vi "Settings UI.vi"(10 "Alias":string, 11 "Init Settings In":T1={"Step Values"=[], "Only Execute When Test Running"=TRUE, "Reset Sequence When Test Starts"=TRUE, "Current Sequence ID"=0, "Total Iterations"=0, "Current Step Start Timestamp"=0.0, "Number of Sequence Steps"=0, "Num of Analog Channels"=0, "Num of Digital Channels"=0, "Delay Before Starting Sequence"=0.0, "Show UI"=FALSE, "Time Remaining"=0.0, "Test Running"=FALSE, "Pause Timestamp"=0.0, "Default Analog Values"=[], "Default Digital Values"=[]}) -> (2 "Applied Settings":T1={"Step Values"=[], "Only Execute When Test Running"=TRUE, "Reset Sequence When Test Starts"=TRUE, "Current Sequence ID"=0, "Total Iterations"=0, "Current Step Start Timestamp"=0.0, "Number of Sequence Steps"=0, "Num of Analog Channels"=0, "Num of Digital Channels"=0, "Delay Before Starting Sequence"=0.0, "Show UI"=FALSE, "Time Remaining"=0.0, "Test Running"=FALSE, "Pause Timestamp"=0.0, "Default Analog Values"=[], "Default Digital Values"=[]}, 3 "Show UI":bool)   [LabVIEW 2020, in "Sequencer with Output Values.lvlib" / "Sequencer with Output Values.lvclass"]
uses:
  Sequencer with Output Values.lvclass
  Params.ctl
  Step Settings.ctl
  Tree Manager/Tree Manager Mode.ctl
  Tree Manager/Control Refs.ctl
  Global Strings.vi
panel:
  in  "Tab Control":enum32{"Numeric", "String", "Bool", "Enum"}(tab)
  in  "Numeric":dbl min=1.0 max=100.0 step=1.0
  in  "String":string
  in  "Boolean":u16(ring) items=["False", "True"]
  in  "Ring":u16(ring) items=["Wait for end of step", "Repeat channel values"]
  in  "Plot Visible Array":cluster{"Boolean 2":bool}[](array[cluster]) caption="Show"
  in  "Applied Settings Control":T1={"Step Values"=[], "Only Execute When Test Running"=TRUE, "Reset Sequence When Test Starts"=TRUE, "Current Sequence ID"=0, "Total Iterations"=0, "Current Step Start Timestamp"=0.0, "Number of Sequence Steps"=0, "Num of Analog Channels"=0, "Num of Digital Channels"=0, "Delay Before Starting Sequence"=0.0, "Show UI"=FALSE, "Time Remaining"=0.0, "Test Running"=FALSE, "Pause Timestamp"=0.0, "Default Analog Values"=[], "Default Digital Values"=[]}
  out "Current Settings":T1={"Step Values"=[], "Only Execute When Test Running"=TRUE, "Reset Sequence When Test Starts"=TRUE, "Current Sequence ID"=0, "Total Iterations"=0, "Current Step Start Timestamp"=0.0, "Number of Sequence Steps"=0, "Num of Analog Channels"=0, "Num of Digital Channels"=0, "Delay Before Starting Sequence"=0.0, "Show UI"=FALSE, "Time Remaining"=0.0, "Test Running"=FALSE, "Pause Timestamp"=0.0, "Default Analog Values"=[], "Default Digital Values"=[]}
  in  "Close":bool
  in  "Apply":bool
  out "Channel Values Preview":waveform(dbl)[](graph)
  out "Setting Description":string
  in  "Settings Tree":string(tree) caption="Settings"
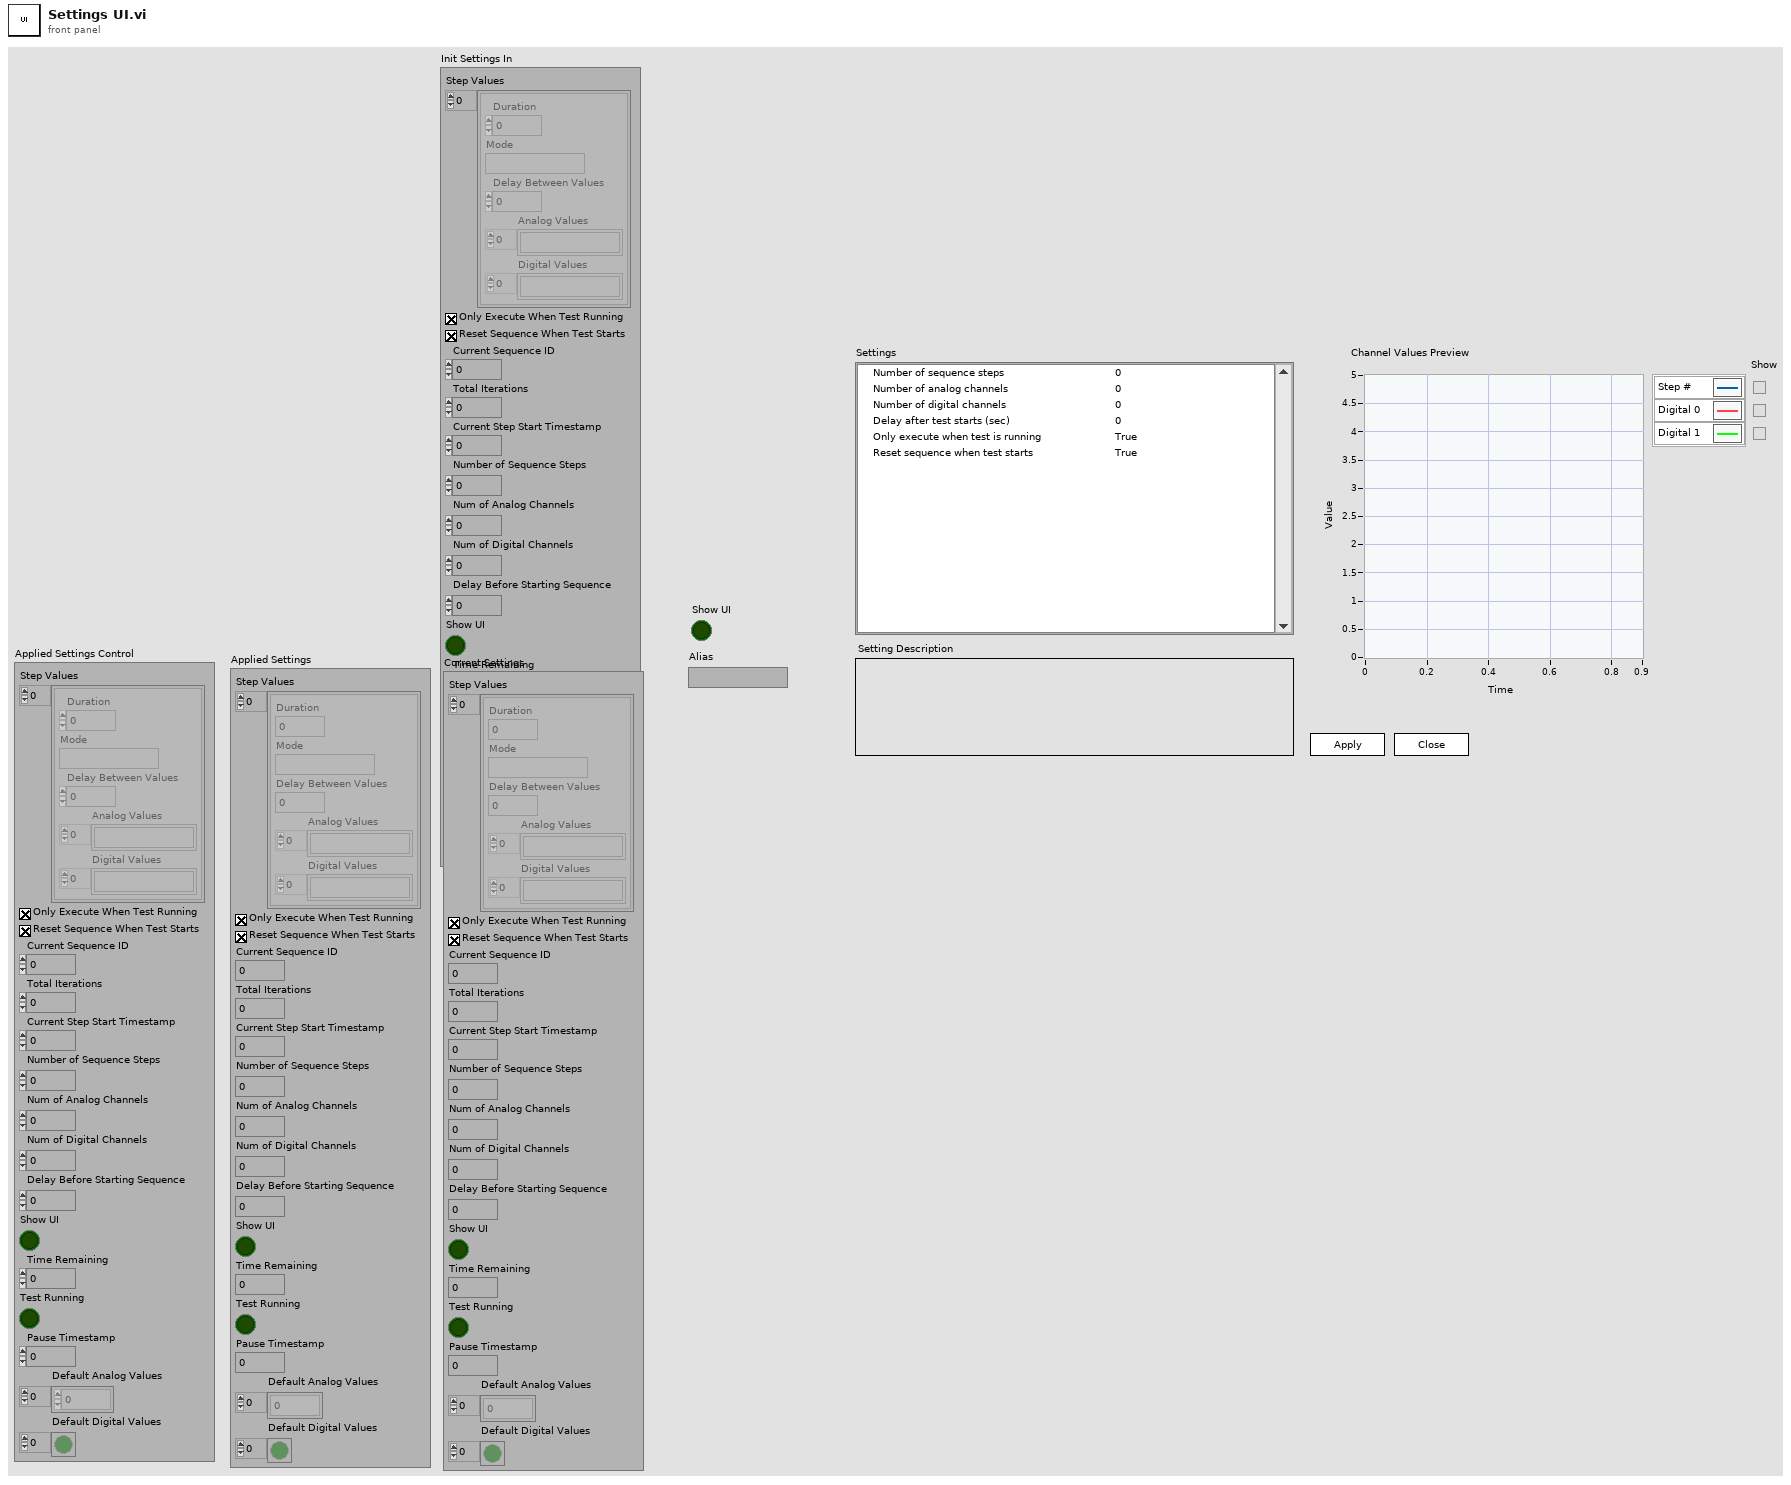
[diagram p1: front panel]
types:
  T1 = typedef "Sequencer with Output Values.lvlib/Sequencer with Output Values.lvclass/Params.ctl" = cluster{"Step Values":T2[], "Only Execute When Test Running":bool, "Reset Sequence When Test Starts":bool, "Current Sequence ID":u32, "Total Iterations":u32, "Current Step Start Timestamp":dbl, "Number of Sequence Steps":i32, "Num of Analog Channels":i32, "Num of Digital Channels":i32, "Delay Before Starting Sequence":dbl, "Show UI":bool, "Time Remaining":dbl, "Test Running":bool, "Pause Timestamp":dbl, "Default Analog Values":dbl[], "Default Digital Values":bool[]}
  T2 = typedef "Sequencer with Output Values.lvlib/Sequencer with Output Values.lvclass/Step Settings.ctl" = cluster{"Duration":dbl, "Mode":string, "Delay Between Values":dbl, "Analog Values":string[], "Digital Values":string[]}
  T3 = cluster{"Numeric":dbl, "String":string, "Boolean":u16, "Ring":u16}
  T4 = typedef "Sequencer with Output Values.lvlib/Sequencer with Output Values.lvclass/Control Refs.ctl" = cluster{"Tree Ref":refnum<vi>, "Tab Control":refnum<vi>, "Numeric":refnum<vi>, "String":refnum<vi>, "Boolean":refnum<vi>, "Enum":refnum<vi>, "Description":refnum<vi>}
  T5 = typedef "Sequencer with Output Values.lvlib/Sequencer with Output Values.lvclass/Tree Manager Mode.ctl" = enum16{"Init", "Tree Change", "Value Change", "Close"}
  T6 = enum32{"Invalid", "Standard", "Closed", "Hidden", "Minimized", "Maximized"}
  T7 = typedef "LVNodeAndColumnTypeDef.ctl" = cluster{"Node":string, "Column":i32}
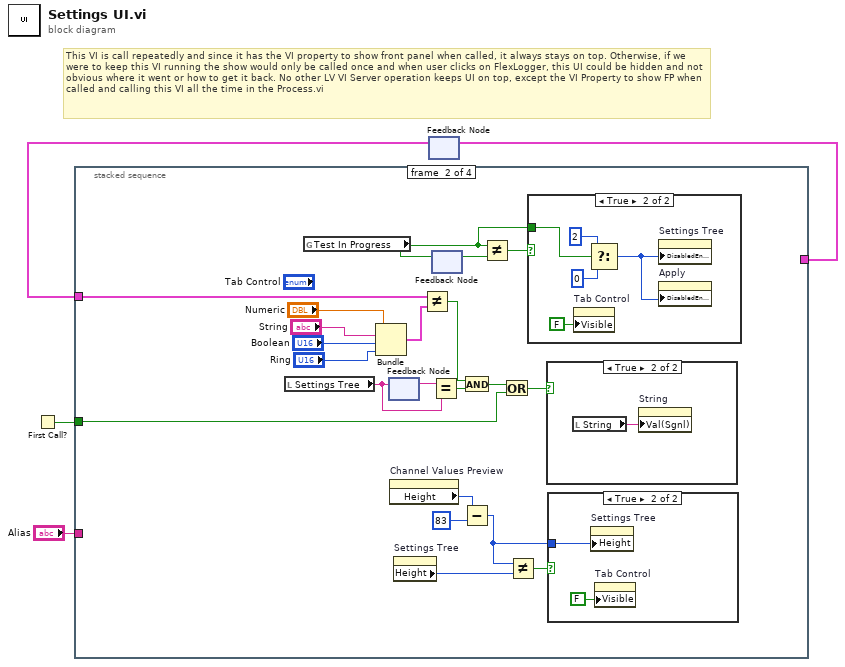
[diagram p0: block diagram]
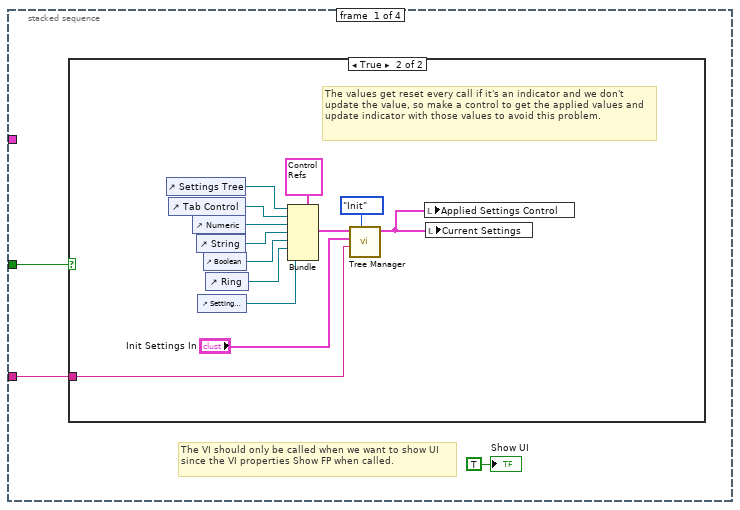
[diagram p2: hidden frame]
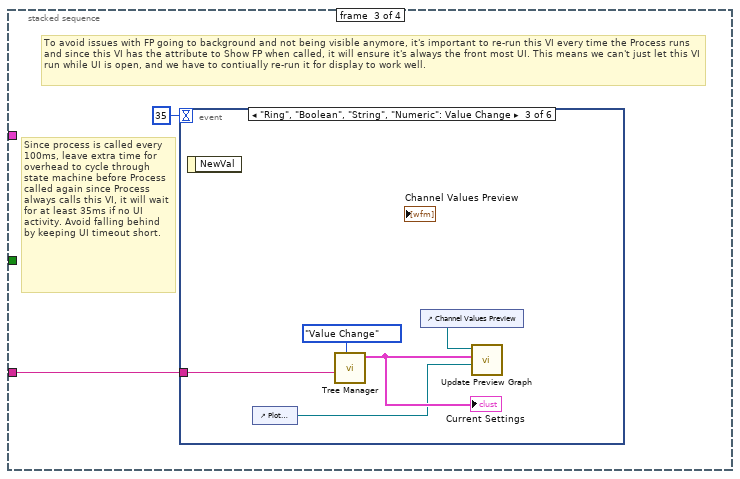
[diagram p7: hidden frame]
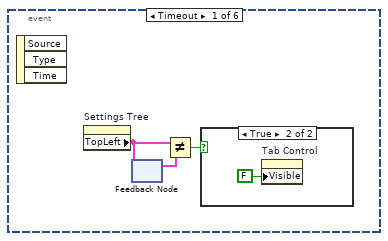
[diagram p8: hidden frame]
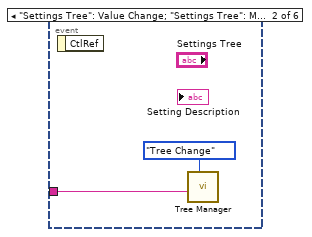
[diagram p10: hidden frame]
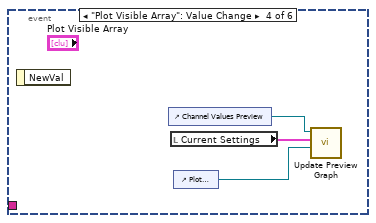
[diagram p11: hidden frame]
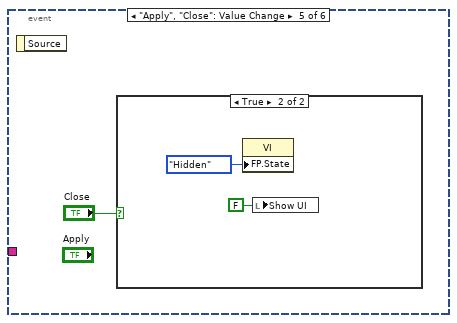
[diagram p12: hidden frame]
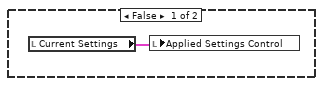
[diagram p13: hidden frame]
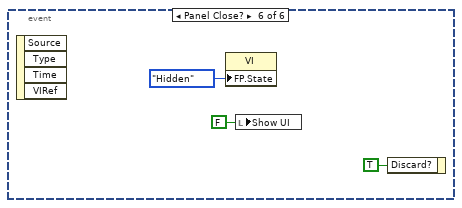
[diagram p14: hidden frame]
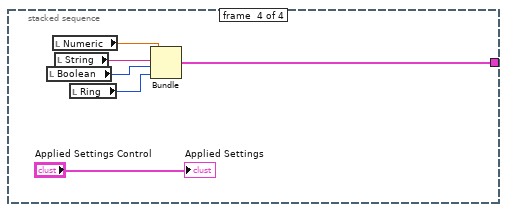
[diagram p15: hidden frame]
diagram:
  # "This VI is call repeatedly and since it has the VI property to show front panel when called, it always stays on top. Otherwise, if we were to keep this VI running the show would only be called once and when user clicks on FlexLogger, this UI could be hidden and not obvious where it went or how to get it back. No other LV VI Server operation keeps UI on top, except the VI Property to show FP when called and calling this VI all the time in the Process.vi"
  n1 = First Call?() -> (First Call?: T/F=w1:bool)
  n2 = feedback #1() -> (w2:T3)  [unwired: 1 in]
  n3 = stacked-sequence {
    tunnel: w1 -> [w6 w31 _ _]
    tunnel: "Alias" -> [w7 _ w50 _]
    tunnel: [_ _ _ w74] -> w3
    tunnel: w2 -> [_ w32 _ _]
    frame #0 {
      # "The VI should only be called when we want to show UI since the VI properties Show FP when called."
      n4 = case shown="True" w6 {
        tunnel: w7 -> [_ w20]
        frame False {
        }
        frame True {
          # "The values get reset every call if it's an indicator and we don't update the value, so make a control to get the applied values and update indicator with those values to avoid this problem."
          n5 = control-ref of="Settings Tree"() -> (w18:refnum<vi>)
          n6 = control-ref of="Tab Control"() -> (w17:refnum<vi>)
          n7 = control-ref of="Numeric"() -> (w16:refnum<vi>)
          n8 = control-ref of="String"() -> (w15:refnum<vi>)
          n9 = control-ref of="Setting Description"() -> (w12:refnum<vi>)
          n10 = control-ref of="Boolean"() -> (w14:refnum<vi>)
          n11 = control-ref of="Ring"() -> (w13:refnum<vi>)
          n12 = Bundle(cluster=T4 {"Tree Ref"=refnum, "Tab Control"=refnum, "Numeric"=refnum, "String"=refnum, "Boolean"=refnum, "Enum"=refnum, "Description"=refnum} ("Init Refs"), "Tree Ref"=w18, "Tab Control"=w17, "Numeric"=w16, "String"=w15, "Boolean"=w14, "Enum"=w13, "Description"=w12) -> (w19:T4)
          n13 = call "Tree Manager.vi"("Mode"=Tree_Manager_Mode."Init", "Alias"=w20, "Init Settings In"="Init Settings In", "Init Refs"=w19) -> ("Settings Out"=w8:T1)  [unwired: 7 in]
          n14 = local write "Applied Settings Control"(w8) -> ()
          n15 = local write "Current Settings"(w8) -> ()
        }
      }
      "Show UI" <- TRUE ("Show UI")
    }
    frame #1 {
      n16 = local read "Settings Tree"() -> (w34:string)
      n17 = global read "Global Strings.vi" "Test In Progress"() -> (w21:bool)
      n18 = Bundle("Numeric"="Numeric", "String"="String", "Boolean"="Boolean", "Ring"="Ring") -> (w41:T3)  [unwired: 1 in]
      n19 = feedback #2() -> (w33:string)  [unwired: 1 in]
      n20 = feedback-in #2(w34) -> ()
      n21 = property on="Channel Values Preview" class="WFGraph (strict)"() -> ("Height"=w28:u32)  [unwired: 2 in, 2 out]
      n22 = property on="Settings Tree" class="Tree (strict)"() -> ("Height"=w26:u32)  [unwired: 2 in, 2 out]
      n23 = Not Equal?(x=w32, y=w41) -> (x != y?=w36:bool)
      n24 = Equal?(x=w33, y=w34) -> (x = y?=w35:bool)
      n25 = feedback #3() -> (w23:bool)  [unwired: 1 in]
      n26 = feedback-in #3(w21) -> ()
      n27 = And(x=w36, y=w35) -> (x .and. y?=w30:bool)
      n28 = Subtract(x=w28, y=u32 83) -> (x-y=w24:u32)
      n29 = Not Equal?(x=w21, y=w23) -> (x != y?=w22:bool)
      n30 = Or(x=w30, y=w31) -> (x .or. y?=w29:bool)
      n31 = Not Equal?(x=w24, y=w26) -> (x != y?=w25:bool)
      n32 = case shown="True" w22 {
        tunnel: w21 -> [_ w46]
        frame False {
        }
        frame True {
          n33 = property on="Tab Control" class="TabCtl (strict)"("Visible"=FALSE) -> ()  [unwired: 2 in, 2 out]
          n34 = Select(t=2, s=w46, f=0) -> (s? t:f=w43:i32)
          n35 = property on="Settings Tree" class="Tree (strict)"("DisabledEnum"=w43) -> ()  [unwired: 2 in, 2 out]
          n36 = property on="Apply" class="Bool"("DisabledEnum"=w43) -> ()  [unwired: 2 in, 2 out]
        }
      }
      n37 = case shown="True" w29 {
        frame False {
        }
        frame True {
          n38 = local read "String"() -> (w49:string)
          n39 = property on="String" class="Str"("Val(Sgnl)"=w49) -> ()  [unwired: 2 in, 2 out]
        }
      }
      n40 = case shown="True" w25 {
        tunnel: w24 -> [_ w48]
        frame False {
        }
        frame True {
          n41 = property on="Settings Tree" class="Tree (strict)"("Height"=w48) -> ()  [unwired: 2 in, 2 out]
          n42 = property on="Tab Control" class="TabCtl (strict)"("Visible"=FALSE) -> ()  [unwired: 2 in, 2 out]
        }
      }
    }
    frame #2 {
      # "Since process is called every 100ms, leave extra time for overhead to cycle through state machine before Process called again since Process always calls this VI, it will wait for at least 35ms if no UI activity. Avoid falling behind by keeping UI timeout short."
      # "To avoid issues with FP going to background and not being visible anymore, it's important to re-run this VI every time the Process runs and since this VI has the attribute to Show FP when called, it will ensure it's always the front most UI. This means we can't just let this VI run while UI is open, and we have to contiually re-run it for display to work well."
      n43 = event shown="[2] \"Ring\", \"Boolean\", \"String\", \"Numeric\": Value Change" {
        selector: _ -> [_ _ _ _ _ _]
        dyn-events: _ -> [_ _ _ _ _ _]
        timeout: 35 -> [_ _ _ _ _ _]
        tunnel: w50 -> [_ w56 w59 _ _ _]
        event Timeout {
          n44 = event-data() -> ()  [unwired: 1 in, 3 out]
          n45 = property on="Settings Tree" class="Tree (strict)"() -> ("TopLeft"=w54:T7)  [unwired: 2 in, 2 out]
          n46 = feedback-in #4(w54) -> ()
          n47 = feedback #4() -> (w53:T7)  [unwired: 1 in]
          n48 = Not Equal?(x=w54, y=w53) -> (x != y?=w52:bool)
          n49 = case shown="True" w52 {
            frame False {
            }
            frame True {
              n50 = property on="Tab Control" class="TabCtl (strict)"("Visible"=FALSE) -> ()  [unwired: 2 in, 2 out]
            }
          }
        }
        event "Settings Tree": Value Change; "Settings Tree": Mouse Down {
          n51 = event-data() -> ()  [unwired: 1 in, 1 out]
          n52 = call "Tree Manager.vi"("Mode"=Tree_Manager_Mode."Tree Change", "Alias"=w56) -> ()  [unwired: 9 in, 1 out]
        }
        event "Ring", "Boolean", "String", "Numeric": Value Change {
          n53 = event-data() -> ()  [unwired: 1 in, 1 out]
          n54 = control-ref of="Plot Visible Array"() -> (w58:refnum<vi>)
          n55 = call "Tree Manager.vi"("Mode"=Tree_Manager_Mode."Value Change", "Alias"=w59) -> ("Settings Out"=w61:T1)  [unwired: 9 in]
          "Current Settings" <- w61
          n56 = control-ref of="Channel Values Preview"() -> (w60:refnum<vi>)
          n57 = call "Update Preview Graph.vi"("Plot Visible Array"=w58, "Settings In"=w61, "Graph Preview Ref"=w60) -> ()  [unwired: 9 in]
        }
        event "Plot Visible Array": Value Change {
          n58 = event-data() -> ()  [unwired: 1 in, 1 out]
          n59 = control-ref of="Channel Values Preview"() -> (w64:refnum<vi>)
          n60 = local read "Current Settings"() -> (w65:T1)
          n61 = control-ref of="Plot Visible Array"() -> (w63:refnum<vi>)
          n62 = call "Update Preview Graph.vi"("Plot Visible Array"=w63, "Settings In"=w65, "Graph Preview Ref"=w64) -> ()  [unwired: 9 in]
        }
        event "Apply", "Close": Value Change {
          n63 = event-data() -> ()  [unwired: 1 in, 1 out]
          n64 = case shown="True" "Close" {
            frame False {
              n65 = local read "Current Settings"() -> (w67:T1)
              n66 = local write "Applied Settings Control"(w67) -> ()
            }
            frame True {
              n67 = property class="VI"("FP.State"=T6."Hidden" ("Front Panel Window:State")) -> ()  [unwired: 2 in, 2 out]
              n68 = local write "Show UI"(FALSE ("Show UI")) -> ()
            }
          }
        }
        event Panel Close? {
          n69 = event-data() -> ()  [unwired: 1 in, 4 out]
          n70 = property class="VI"("FP.State"=T6."Hidden" ("Front Panel Window:State")) -> ()  [unwired: 2 in, 2 out]
          n71 = local write "Show UI"(FALSE ("Show UI")) -> ()
          n72 = event-data("Discard?"=TRUE) -> ()  [unwired: 1 in, 1 out]
        }
      }
    }
    frame #3 {
      n73 = local read "Boolean"() -> (w77:u16)
      n74 = local read "Numeric"() -> (w75:dbl)
      n75 = local read "String"() -> (w76:string)
      n76 = local read "Ring"() -> (w78:u16)
      n77 = Bundle("Numeric"=w75, "String"=w76, "Boolean"=w77, "Ring"=w78) -> (w74:T3)  [unwired: 1 in]
      "Applied Settings" <- "Applied Settings Control"
    }
  }
  n78 = feedback-in #1(w3) -> ()
